vi "MN logic.vi"(0 "Total Count":u64, 5 "Fail Count Array In":u64[](array[numeric]), 7 "M":u8, 9 "N":u64, 11 "error in (no error)":errorcluster) -> (4 "Result Out":bool, 6 "Fail Count Array Out":u64[](array[numeric]), 15 "error out":errorcluster)   [LabVIEW 2019, in "Rack Controller.lvclass"]
uses:
  Rack Controller.lvclass
panel:
  out "End Count":u64
  out "In Range?":bool
  out "Start Count":u64
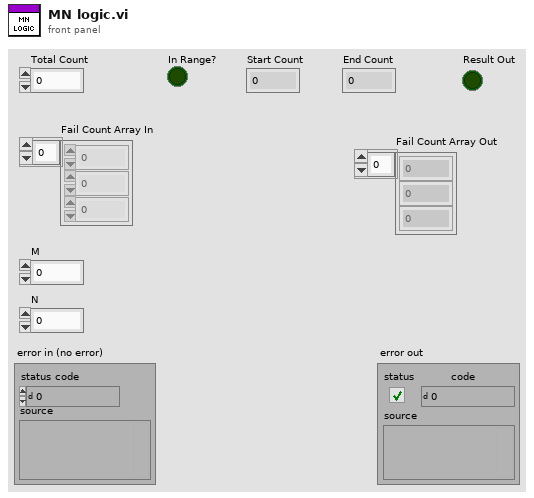
[diagram p1: front panel]
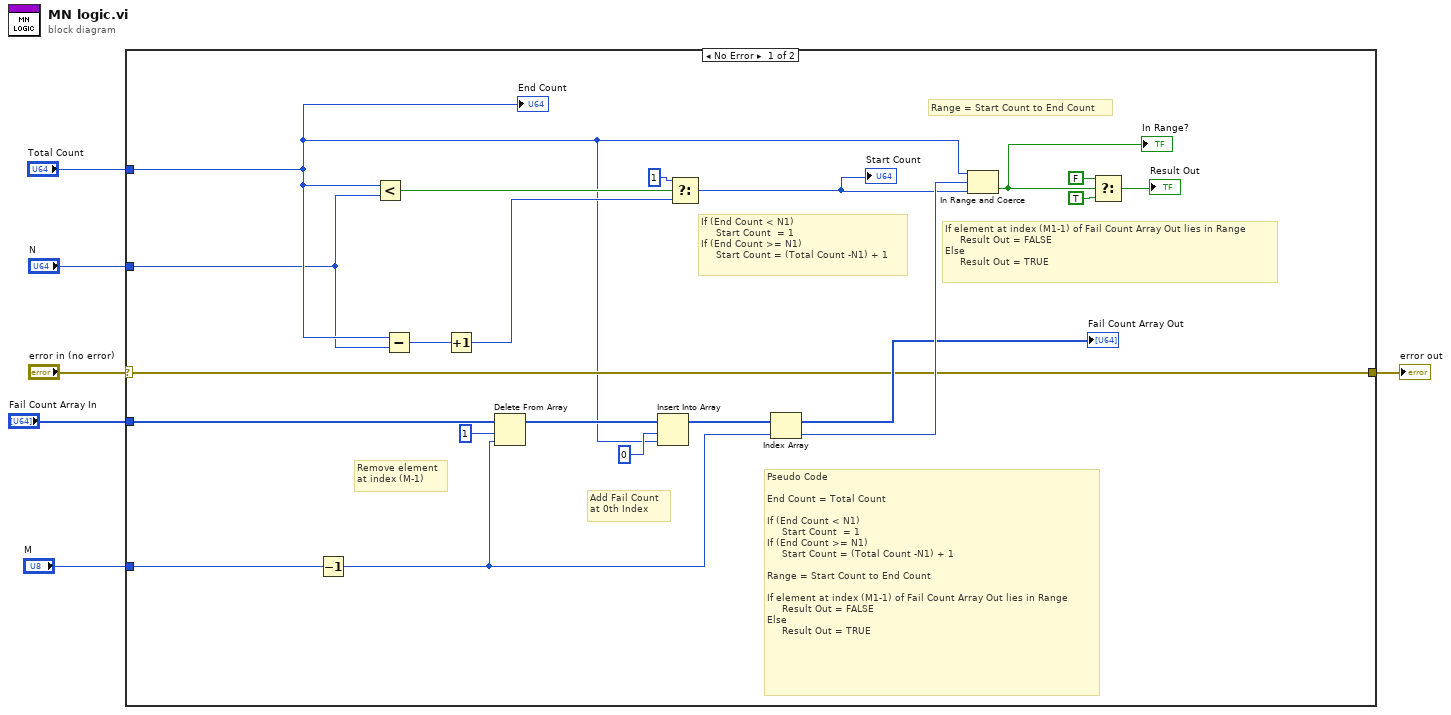
[diagram p0: block diagram]
diagram:
  n1 = case shown="No Error" "error in (no error)" {
    selector: "error in (no error)" -> [w13 w27]
    tunnel: [w13 w27] -> w5
    tunnel: "Total Count" -> [w12 _]
    tunnel: "N" -> [w11 _]
    tunnel: "Fail Count Array In" -> [w10 _]
    tunnel: "M" -> [w9 _]
    frame No Error {
      # "Add Fail Count\nat 0th Index"
      # "Remove element\nat index (M-1)"
      # "If element at index (M1-1) of Fail Count Array Out lies in Range\n     Result Out = FALSE \nElse\n     Result Out = TRUE"
      # "Range = Start Count to End Count"
      # "If (End Count < N1)\n     Start Count  = 1\nIf (End Count >= N1)\n     Start Count = (Total Count -N1) + 1"
      # "Pseudo Code\n\nEnd Count = Total Count\n\nIf (End Count < N1)\n     Start Count  = 1\nIf (End Count >= N1)\n     Start Count = (Total Count -N1) + 1 \n\nRange = Start Count to End Count\n\nIf element at index (M1-1) of Fail Count Array Out lies in Range\n     Result Out = FALSE \nElse\n     Result Out = TRUE"
      n2 = Decrement(x=w9) -> (x-1=w18:u8)
      n3 = Less?(x=w12, y=w11) -> (x < y?=w26:bool)
      n4 = Subtract(x=w12, y=w11) -> (x-y=w24:u64)
      n5 = Increment(x=w24) -> (x+1=w23:u64)
      n6 = Delete From Array "Delete From Array"(array=w10, length=1, index=w18) -> (array with subset deleted=w16:u64[])  [unwired: 1 out]
      n7 = Insert Into Array "Insert Into Array"(array=w16, index=0, new element=w12) -> (w14:u64[])
      "Fail Count Array Out" <- w14
      n8 = Select(t=u64 1, s=w26, f=w23) -> (s? t:f=w21:u64)
      "Start Count" <- w21
      n9 = Index Array "Index Array"(array=w14, index=w18) -> (element=w22:u64)
      n10 = In Range and Coerce(upper limit=w12, x=w22, lower limit=w21) -> (In Range?=w8:bool)  [unwired: 1 out]
      "In Range?" <- w8
      n11 = Select(t=FALSE, s=w8, f=TRUE) -> (s? t:f=→"Result Out":bool)
      "End Count" <- w12
    }
    frame Error {
    }
  }
  "error out" <- w5
